vi "Set Callback On Visible Frame Init.vi"(10 "OnVisibleFrameInit":cluster{}, 11 "index":u16) -> (3 "function return":i32)   [LabVIEW 2025, in "ExtremelyEpicImagerIPC2.lvlib"]
doc: "IMAGERIPC_API HRESULT WINAPI SetCallback_OnVisibleFrameInit(WORD index, fpOnFrameInit OnVisibleFrameInit);"
uses:
  ExtremelyEpicImagerIPC2.lvlib
  ImagerIPC2.dll
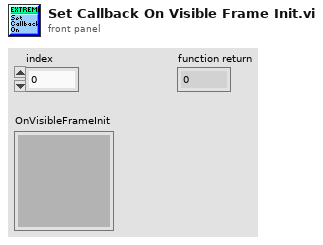
[diagram p1: front panel]
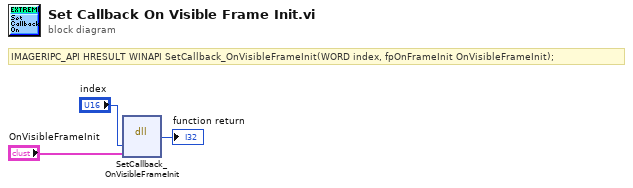
[diagram p0: block diagram]
diagram:
  # "IMAGERIPC_API HRESULT WINAPI SetCallback_OnVisibleFrameInit(WORD index, fpOnFrameInit OnVisibleFrameInit);"
  n1 = dll-call lib="C:/Users/mayhe/OneDrive/Documents/GitHub/In-situ-monitoring-of-powder-bed-fusion-additive-manufacturing/system_development/Orichalcum/v0.2/Software_design/thermal-camera/VI/Connect SDK/ImagerIPC2.*" fn="SetCallback_OnVisibleFrameInit"("index"="index", "OnVisibleFrameInit"="OnVisibleFrameInit") -> (→"function return":i32)  [unwired: 5 in, 2 out]
